vi "DesignEngineINI.vi"() -> (0 "Ini file path":path=path "C:/ProgramData/Design Engine/Design Engine.ini", 3 "Application Name":string="Design Engine")   [LabVIEW 2015, in "Design Server.lvlib"]
uses:
  Design Server.lvlib
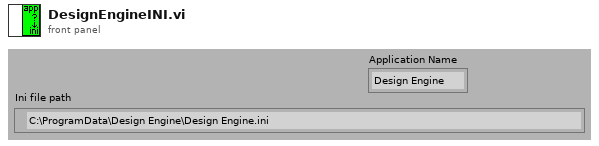
[diagram p1: front panel]
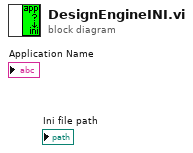
[diagram p0: block diagram]
diagram:
